vi "Buffered Read, My version.vi"() -> ()   [LabVIEW 2010]
panel:
  out "Waveform Chart":u16[](graph)
  out "Error Code":i32
  out "Error Message":string
  in  "InterChannel Delay":sgl=-1.0 format="%.2f"
  in  "Range":i32(ring)=1 items=["Not Programmable"=0, "+- 20 V"=27, "+- 10 V"=1, "+- 5 V"=2, "+- 4 V"=28, "+- 2.5 V"=3, "+- 2 V"=29, "+- 1.67 V"=4, "+- 1.25 V"=5, "+- 1 V"=6, "+- .625 V"=7, "+- .5 V"=8, "+- .25 V"=30, "+- .2 V"=31, "+- .1 V"=9, "+- .05 V"=10, "+- .01 V"=11, "+- .005 V"=12, "0 - 10 V"=13, "0 - 5 V"=14, "0 - 4 V"=36, "0 - 2.5 V"=15, "0 - 2 V"=16, "0 - 1.67 V"=17, "0 - 1.25 V"=18, "0 - 1 V"=19, "0 - .5 V"=32, "0 - .25 V"=33, "0 - .2 V"=34, "0 - .1 V"=20, "0 - .02 V"=35, "0 - .01 V"=21, "4 - 20 mA"=22, "2 - 10 mA"=23, "1 - 5 mA"=24, ".5 - 2.5 mA"=25, "0 - 20 mA"=26]
  in  "Options":i32
  in  "Rate":i32
  in  "Count":i32
  in  "Low Channel":i32
  in  "High Channel":i32
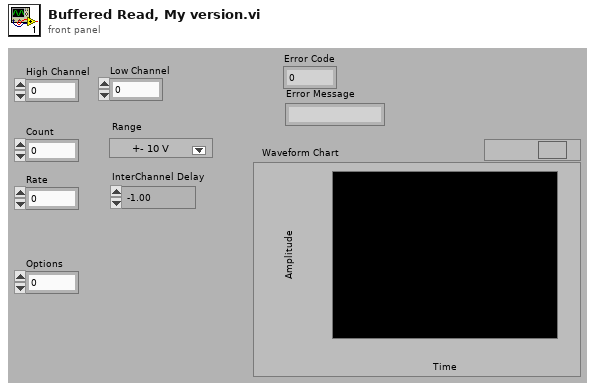
[diagram p1: front panel]
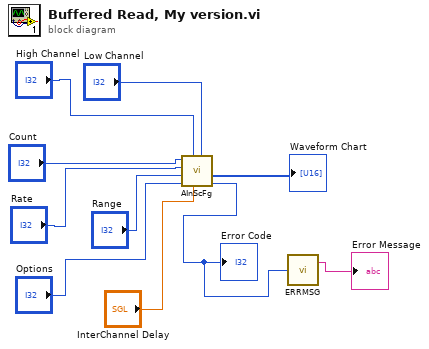
[diagram p0: block diagram]
diagram:
  n1 = call <menus>:"AInScFg.VI"("LowChan"="Low Channel", "InterChannel Delay"="InterChannel Delay", "HighChan"="High Channel", "Options"="Options", "Range"="Range", "Rate"="Rate", "Count"="Count") -> ("ErrCode"=w10:i32, "ADData"=→"Waveform Chart":u16[])  [unwired: 1 in, 1 out]
  "Error Code" <- w10
  n2 = call <menus>:"ERRMSG.VI"("ErrCode"=w10) -> ("ErrMsg"=→"Error Message":string)  [unwired: 1 out]
